vi "Test_LaunchActors_NestedError_CallerReceivesError.vi"(8 "error in (no error)":errorcluster, 11 "TestCase in":refnum<class "TestLaunchAndShutdown.lvclass">) -> (0 "error out":errorcluster, 3 "TestCase out":refnum<class "TestLaunchAndShutdown.lvclass">)   [LabVIEW 2017, in "TestLaunchAndShutdown.lvclass"]
uses:
  TestLaunchAndShutdown.lvclass
  Doubles/ActorGeneratesError/ActorGeneratesError.lvclass
  C:/Program Files (x86)/National Instruments/LabVIEW 2017/vi.lib/ActorFramework/Actor/Actor.lvclass
  Doubles/ActorNotifiesWhenStopped/ActorNotifiesWhenStopped.lvclass
  <vilib>/ActorFramework/Actor/Actor.lvclass
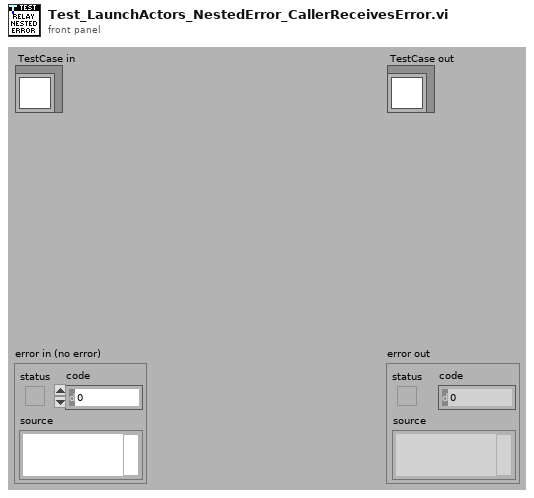
[diagram p1: front panel]
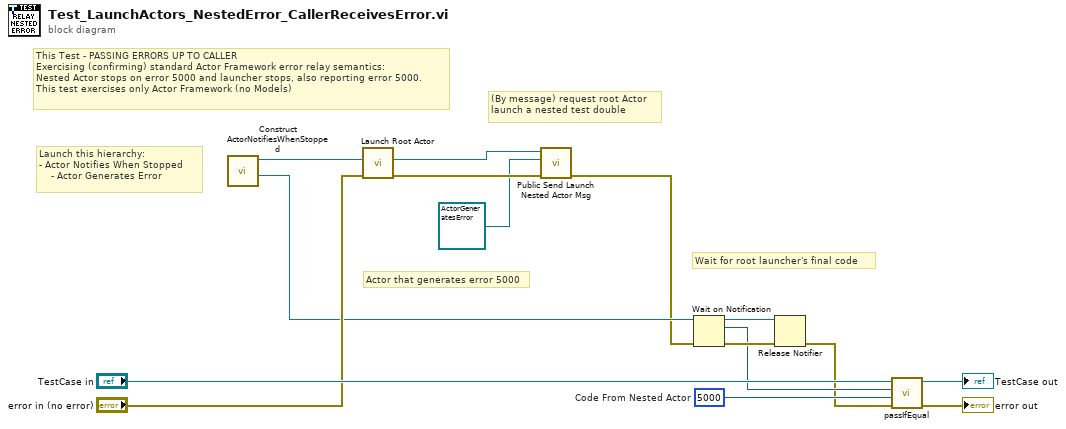
[diagram p0: block diagram]
diagram:
  w2 = 5000  # Code From Nested Actor
  # "(By message) request root Actor\nlaunch a nested test double"
  # "Wait for root launcher's final code"
  # "This Test - PASSING ERRORS UP TO CALLER\nExercising (confirming) standard Actor Framework error relay semantics:\nNested Actor stops on error 5000 and launcher stops, also reporting error 5000.\nThis test exercises only Actor Framework (no Models)"
  # "Actor that generates error 5000"
  # "Launch this hierarchy:\n- Actor Notifies When Stopped\n    - Actor Generates Error"
  n1 = call "Construct ActorNotifiesWhenStopped.vi"() -> ("Final Error Notifier"=w11:refnum<notifier>, "RootModelNotifiesWhenStopped out"=w7:refnum<class "ActorNotifiesWhenStopped.lvclass">)  [unwired: 10 in]
  n2 = call <vilib>:"Launch Root Actor.vi"("error in (no error)"="error in (no error)", "Actor"=w7) -> ("error out"=w10:errorcluster, "Actor's Enqueuer"=w6:refnum<class "Message Enqueuer.lvclass">)  [unwired: 8 in]
  n3 = call "Public Send Launch Nested Actor Msg.vi"("error in"=w10, "Nested Actor"=refnum<class "ActorGeneratesError.lvclass"> refnum ("ActorGeneratesError.lvclass"), "Self Enqueuer in"=w6) -> ("error out"=w4:errorcluster)  [unwired: 7 in, 1 out]
  n4 = Wait on Notification(notifier=w11, error in (no error)=w4) -> (notifier out=w8:refnum<notifier>, notification=w3:i32, error out=w9:errorcluster)  [unwired: 2 in, 1 out]
  n5 = Release Notifier(notifier=w8, error in (no error)=w9) -> (error out=w1:errorcluster)  [unwired: 1 in, 2 out]
  n6 = call-dynamic "passIfEqual.vi"("error in (no error)"=w1, "y"=w2, "x"=w3, "TestCase in"="TestCase in") -> ("error out"=→"error out":errorcluster, "TestCase out"=→"TestCase out":refnum<class "TestLaunchAndShutdown.lvclass">)  [unwired: 6 in]
